vi "DSF.Engine.Transceiver Thread.Initialize Intermediate Buffers.vi"(8 "error in (no error)":errorcluster, 10 "largest block count":u64, 11 "Transceiver Thread in":refnum<class "DSF.Engine.Transceiver Thread.lvclass">) -> (0 "error out":errorcluster, 3 "Transceiver Thread out":refnum<class "DSF.Engine.Transceiver Thread.lvclass">)   [LabVIEW 2017, in "Data Sharing Framework Engine.lvlib" / "DSF.Engine.Transceiver Thread.lvclass"]
uses:
  DSF.Engine.Transceiver Thread.lvclass
  Shared/Typedefs/DSF Runtime Type Buffers.ctl
  DSF.Engine.Transceiver Thread.lvclass/DSF.Engine.Transceiver Thread.ctl
  Source/Data Sharing Framework Core/Engine/Data Sharing Framework Engine.lvlib
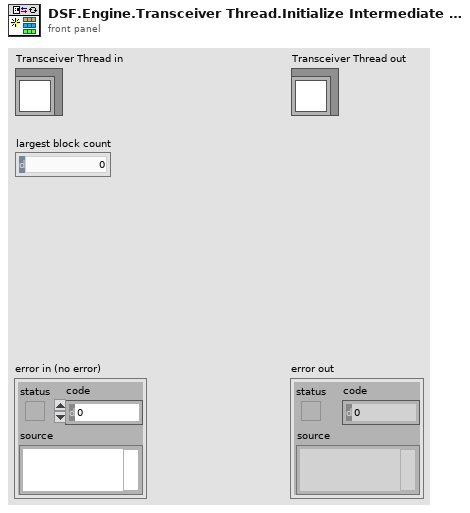
[diagram p1: front panel]
types:
  T1 = typedef "Data Sharing Framework Engine.lvlib/DSF Runtime Type Buffers.ctl" = cluster{"Bool":bool[], "SGL":sgl[], "DBL":dbl[], "I8":i8[], "I16":i16[], "I32":i32[], "I64":i64[], "U8":u8[], "U16":u16[], "U32":u32[], "U64":u64[]}
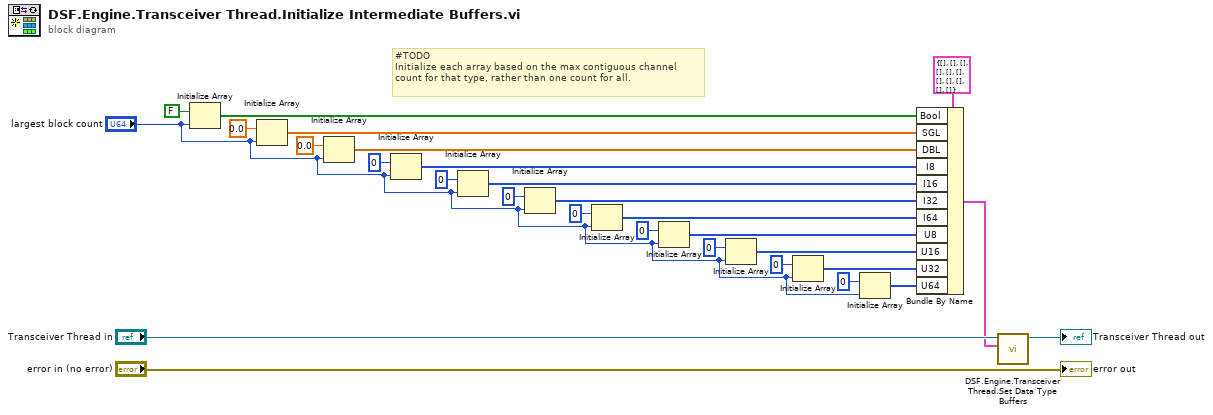
[diagram p0: block diagram]
diagram:
  # "#TODO\nInitialize each array based on the max contiguous channel count for that type, rather than one count for all."
  n1 = Initialize Array(FALSE, "largest block count") -> (w25:bool[])
  n2 = Initialize Array(sgl 0.0, "largest block count") -> (w24:sgl[])
  n3 = Initialize Array(0.0, "largest block count") -> (w21:dbl[])
  n4 = Initialize Array(i8 0, "largest block count") -> (w6:i8[])
  n5 = Initialize Array(i16 0, "largest block count") -> (w7:i16[])
  n6 = Initialize Array(0, "largest block count") -> (w8:i32[])
  n7 = Initialize Array(i64 0, "largest block count") -> (w9:i64[])
  n8 = Initialize Array(u8 0, "largest block count") -> (w10:u8[])
  n9 = Initialize Array(u16 0, "largest block count") -> (w11:u16[])
  n10 = Initialize Array(u32 0, "largest block count") -> (w12:u32[])
  n11 = Initialize Array(u64 0, "largest block count") -> (w13:u64[])
  n12 = Bundle By Name(cluster=T1 {"Bool"=[], "SGL"=[], "DBL"=[], "I8"=[], "I16"=[], "I32"=[], "I64"=[], "U8"=[], "U16"=[], "U32"=[], "U64"=[]} ("Data Type Buffers"), "Bool"=w25, "SGL"=w24, "DBL"=w21, "I8"=w6, "I16"=w7, "I32"=w8, "I64"=w9, "U8"=w10, "U16"=w11, "U32"=w12, "U64"=w13) -> (w1:T1)
  n13 = call "DSF.Engine.Transceiver Thread.Set Data Type Buffers.vi"("data type buffers"=w1, "Transceiver Thread in"="Transceiver Thread in") -> ("Transceiver Thread out"=→"Transceiver Thread out":refnum<class "DSF.Engine.Transceiver Thread.lvclass">)  [unwired: 9 in]
  "error out" <- "error in (no error)"
